vi "DIM_DIO.constructor.vi"(0 "name":string, 2 "data in":string, 5 "error in (no error)":errorcluster) -> (14 "i ref out":refnum<vi>, 16 "data out":string, 19 "error out":errorcluster)   [LabVIEW 2014, in "DIM_DIO.lvlib"]
doc: "constructor of the DIM_DIO class"
uses:
  DIM_DIO.lvlib
  CS_Core/CSApplicationBaseClasses/DeviceBase/DeviceBase.myEventNames.ctl
  CS_Core/CSApplicationBaseClasses/DigiIOBase/DigiIOBase.myEventNames.ctl
  CS_Core/CSSystem/CSSystemLib/CSSystemLib.lvlib
  CSlibraries-extern/DimLVEvent/LVDimInterface/LVDimInterface.lvlib
  CS_Core/CSApplicationBaseClasses/DigiIOBase/DigiIOBase.lvlib
  CS_Core/CSApplicationBaseClasses/DeviceBase/DeviceBase.lvlib
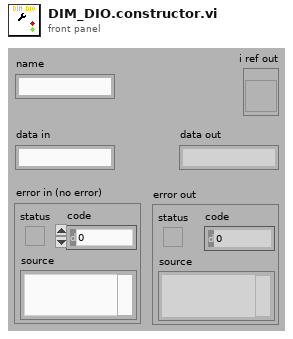
[diagram p1: front panel]
types:
  T1 = enum16{"SetAttribute", "GetAttribute", "CreateAttribute", "DestroyAttribute", "DestroyAllAtributes"}
  T2 = typedef "DigiIOBase.lvlib/DigiIOBase.myEventNames.ctl" = enum16{"lvmsg://SetWord", "lvmsg://GetWord", "lvmsg://SetBit", "lvmsg://GetBit"}
  T3 = typedef "DeviceBase.lvlib/DeviceBase.myEventNames.ctl" = enum16{"lvmsg://Initialize", "lvmsg://Close", "lvmsg://Configure", "lvmsg://Reset", "lvmsg://IDQuery"}
  T4 = typedef "DIM_DIO.lvlib/DIM_DIO.i attribute.ctl" = cluster{"serviceIDs":cluster{"writeBitID":i32}}
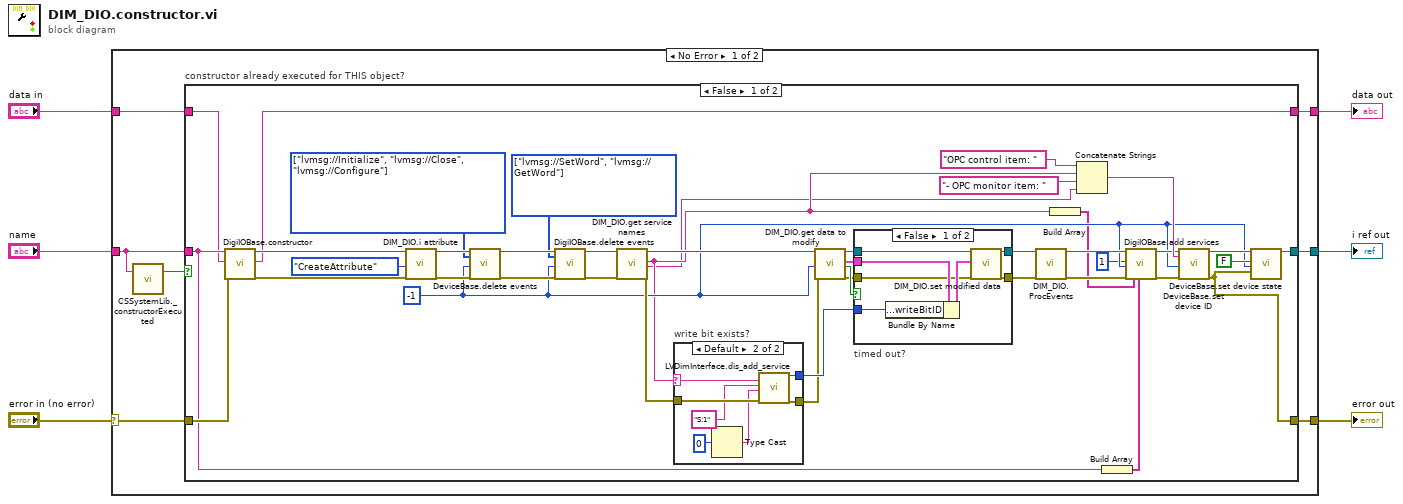
[diagram p0: block diagram]
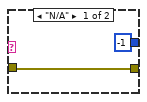
[diagram p3: hidden frame]
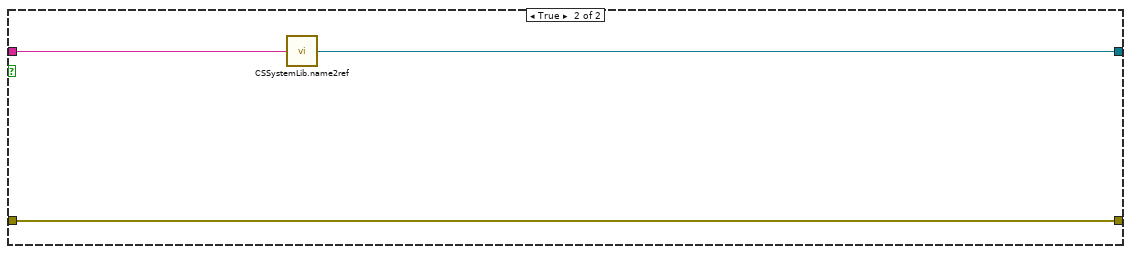
[diagram p4: hidden frame]
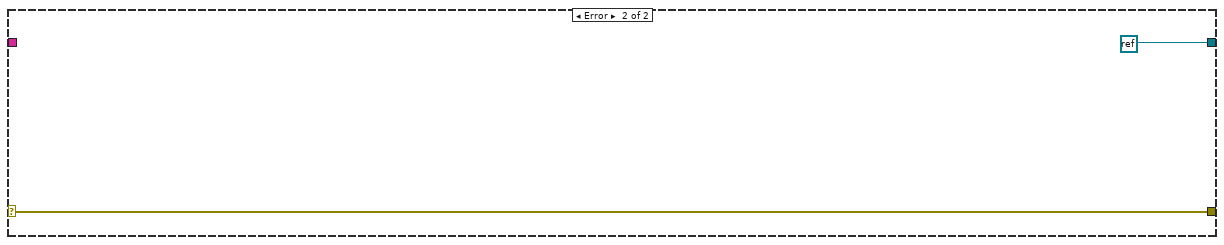
[diagram p5: hidden frame]
diagram:
  n1 = case shown="No Error" "error in (no error)" {
    selector: "error in (no error)" -> [w11 w77]
    tunnel: "name" -> [w10 _]
    tunnel: [w13 refnum<k0> refnum] -> w5
    tunnel: [w12 w77] -> w4
    tunnel: "data in" -> [w8 _]
    tunnel: [w7 _] -> w1
    frame No Error {
      n2 = call "CSSystemLib._constructorExecuted.vi"("name"=w10) -> ("constructor executed?"=w9:bool)  [unwired: 18 in]
      n3 = case "constructor already executed for THIS object?" shown="False" w9 {
        tunnel: [w29 w75] -> w13
        tunnel: [w30 w74] -> w12
        tunnel: w11 -> [w52 w74]
        tunnel: w10 -> [w21 w76]
        tunnel: w8 -> [w15 _]
        tunnel: [w14 _] -> w7
        frame False {
          w37 = T2[] [enum."lvmsg://SetWord", enum."lvmsg://GetWord"] items=["lvmsg://SetWord", "lvmsg://GetWord", "lvmsg://SetBit", "lvmsg://GetBit"] ("events")
          w40 = T3[] [enum."lvmsg://Initialize", enum."lvmsg://Close", enum."lvmsg://Configure"] items=["lvmsg://Initialize", "lvmsg://Close", "lvmsg://Configure", "lvmsg://Reset", "lvmsg://IDQuery"] ("events")
          w24 = -1 ("ms timeout (10000)")
          n4 = call "DigiIOBase.constructor.vi"("name"=w21, "data in"=w15, "error in (no error)"=w52) -> ("i ref out"=w55:refnum<vi>, "data out"=w14:string, "error out"=w54:errorcluster)  [unwired: 14 in]
          n5 = call "DIM_DIO.i attribute.vi"("VI Refnum"=w55, "Action"=T1."CreateAttribute", "error in (no error)"=w54) -> ("VI Refnum out"=w42:refnum<vi>, "error out"=w41:errorcluster)  [unwired: 14 in, 1 out]
          n6 = call "DeviceBase.delete events.vi"("i ref in"=w42, "events"=w40, "ms timeout (10000)"=w24, "error in (no error)"=w41) -> ("i ref out"=w39:refnum<vi>, "error out"=w38:errorcluster)  [unwired: 13 in, 1 out]
          n7 = call "DigiIOBase.delete events.vi"("i ref in"=w39, "events"=w37, "ms timeout (10000)"=w24, "error in (no error)"=w38) -> ("i ref out"=w36:refnum<vi>, "error out"=w35:errorcluster)  [unwired: 13 in, 1 out]
          n8 = call "DIM_DIO.get service names.vi"("i ref in"=w36, "error in (no error)"=w35) -> ("i ref out"=w50:refnum<vi>, "writeService"=w18:string, "readService"=w16:string, "error out"=w51:errorcluster)  [unwired: 14 in]
          n9 = case "write bit exists?" shown="Default" w18 {
            selector: w18 -> [_ w71]
            tunnel: w51 -> [w65 w72]
            tunnel: [w65 w67] -> w43
            tunnel: [-1 w68] -> w45
            frame "N/A" {
            }
            frame Default {
              n10 = Type Cast(x=i16 0) -> (*(type *) &x=w69:string)  [unwired: 1 in]
              n11 = call "LVDimInterface.dis_add_service.vi"("serviceName"=w71, "typeDescriptor"="S:1", "data"=w69, "error in (no error)"=w72) -> ("my_serviceID"=w68:i32, "error out"=w67:errorcluster)  [unwired: 14 in]
            }
          }
          n12 = call "DIM_DIO.get data to modify.vi"("i ref in"=w50, "ms timeout (10000)"=w24, "error in (no error)"=w43) -> ("i ref out"=w48:refnum<vi>, "i attribute"=w47:T4, "timed out"=w49:bool, "error out"=w46:errorcluster)  [unwired: 13 in]
          n13 = case "timed out?" shown="False" w49 {
            tunnel: w48 -> [w62 w64]
            tunnel: w47 -> [w61 _]
            tunnel: w46 -> [w59 w63]
            tunnel: w45 -> [w58 _]
            tunnel: [w57 w63] -> w44
            tunnel: [w56 w64] -> w34
            frame False {
              n14 = Bundle By Name(cluster=w61, "serviceIDs.writeBitID"=w58) -> (w60:T4)
              n15 = call "DIM_DIO.set modified data.vi"("i ref in"=w62, "i attribute"=w60, "error in (no error)"=w59) -> ("i ref out"=w56:refnum<vi>, "error out"=w57:errorcluster)  [unwired: 15 in]
            }
            frame True {
            }
          }
          n16 = call "DIM_DIO.ProcEvents.vi"("i ref in"=w34, "error in (no error)"=w44) -> ("i ref out"=w28:refnum<vi>, "error out"=w26:errorcluster)  [unwired: 16 in]
          n17 = Build Array(w18) -> (w22:string[])
          n18 = Concatenate Strings("OPC control item: " ("string"), w18, "- OPC monitor item: " ("string"), w16) -> (w33:string)
          n19 = Build Array(w21) -> (w20:string[])
          n20 = call "DigiIOBase.add services.vi"("i ref in"=w28, "nofBits"=1, "ms timeout (10000)"=w24, "error in (no error)"=w26, "physicalNames"=w22, "logicalNames"=w20) -> ("i ref out"=w27:refnum<vi>, "error out"=w25:errorcluster)  [unwired: 11 in, 1 out]
          n21 = call "DeviceBase.set device ID.vi"("i ref in"=w27, "deviceID"=w33, "ms timeout (10000)"=w24, "error in (no error)"=w25) -> ("i ref out"=w32:refnum<vi>, "error out"=w30:errorcluster)  [unwired: 13 in, 1 out]
          n22 = call "DeviceBase.set device state.vi"("i ref in"=w32, "implicit"=FALSE, "ms timeout (10000)"=w24, "device error"=w30) -> ("i ref out"=w29:refnum<vi>)  [unwired: 13 in, 2 out]
        }
        frame True {
          n23 = call "CSSystemLib.name2ref.vi"("name"=w76) -> ("obj refnum"=w75:refnum<vi>)
        }
      }
    }
    frame Error {
    }
  }
  "i ref out" <- w5
  "error out" <- w4
  "data out" <- w1
